vi "selectionneur d axe de l accelerometre.vi"(11 "Enum":enum16{"z", "y"}(ring)) -> (2 "VALEUR NUMERIQUE DE L AXE CHOISI":i16)   [LabVIEW 2019]
uses:
  <vilib>/rvi/Emulation/niFpgaSctlEmulationGetInTimedLoop.vi
  <vilib>/rvi/Emulation/niFpgaProcessEmulError.vi
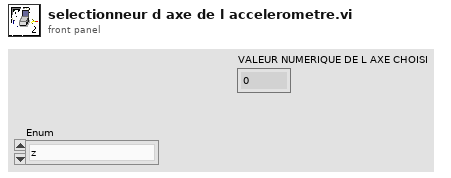
[diagram p1: front panel]
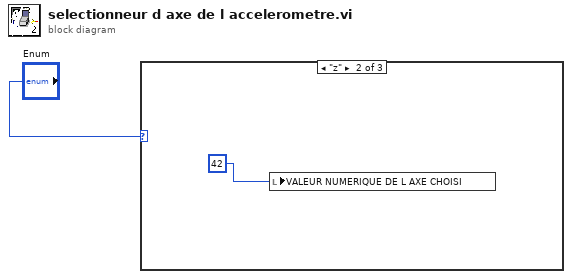
[diagram p0: block diagram]
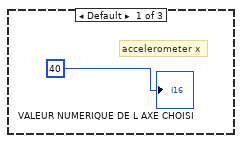
[diagram p2: hidden frame]
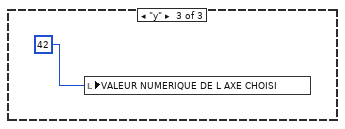
[diagram p3: hidden frame]
diagram:
  n1 = case shown="\"z\"" "Enum" {
    frame Default {
      # "accelerometer x"
      "VALEUR NUMERIQUE DE L AXE CHOISI" <- i16 40
    }
    frame "z" {
      n2 = local write "VALEUR NUMERIQUE DE L AXE CHOISI"(i16 42) -> ()
    }
    frame "y" {
      n3 = local write "VALEUR NUMERIQUE DE L AXE CHOISI"(i16 42) -> ()
    }
  }
